vi "Accel_Read.vi"(8 "error in":errorcluster, 9 "Sensitivity":dbl, 10 "Axis":T3 items=["X-Axis", "Y-Axis", "Z-Axis"], 11 "I2CDevRef":T1 {"Device Address" format="%.0x"}) -> (0 "error out":errorcluster, 2 "Acceleration":dbl, 3 "I2CDevRef Out":T1 {"Device Address" format="%.0x"})   [LabVIEW 2011]
uses:
  Accel_ Axis.ctl
  <vilib>/Rock Robotics/WPI/I2C/WPI_I2CDevRef.ctl
  <vilib>/Rock Robotics/SystemInterfaces/Typedef/FPGA_TypedefDigitalModule.ctl
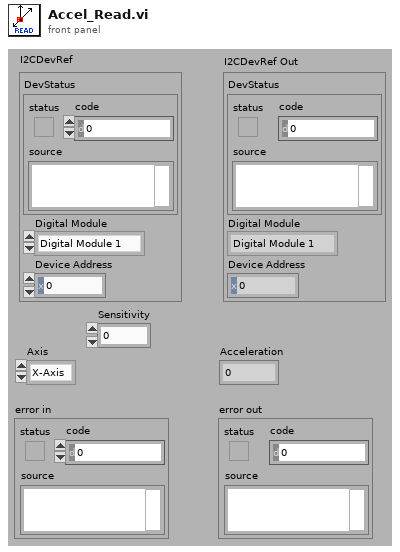
[diagram p1: front panel]
types:
  T1 = typedef "WPI_I2CDevRef.ctl" = cluster{"DevStatus":errorcluster, "Digital Module":T2, "Device Address":u8}
  T2 = typedef "FPGA_TypedefDigitalModule.ctl" = enum16{"Digital Module 1", "Digital Module 2"}
  T3 = typedef "Accel_ Axis.ctl" = u8
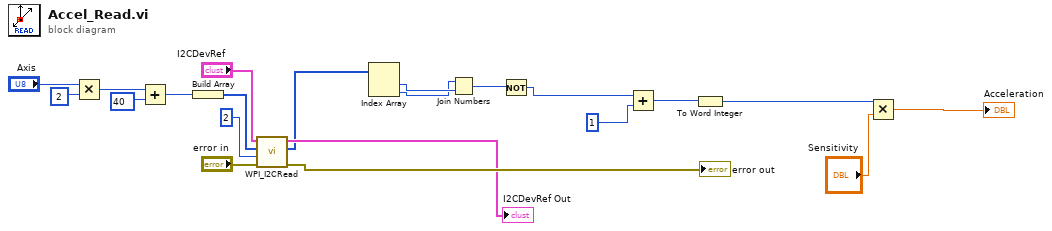
[diagram p0: block diagram]
diagram:
  n1 = Multiply(x="Axis", y=u8 2 ("Data To Send")) -> (x*y=w21:T3)
  n2 = Add(x=w21, y=u8 40 ("Data To Send")) -> (x+y=w11:T3)
  n3 = Build Array(w11) -> (w15:T3[])
  n4 = call <vilib>:"WPI_I2CRead.vi"("error in (no error)"="error in", "I2CBytesToRead"=u8 2, "I2CRegister"=w15, "I2CDevRef"="I2CDevRef") -> ("error out"=→"error out":errorcluster, "Data Out"=w7:u8[], "I2CDevRef"=→"I2CDevRef Out":T1)  [unwired: 1 in, 4 out]
  n5 = Index Array(array=w7) -> (element #1=w6:u8, element #2=w5:u8)  [unwired: 2 in]
  n6 = Join Numbers(hi=w5, lo=w6) -> ((hi.lo)=w4:u16)
  n7 = Not(x=w4) -> (.not. x?=w3:u16)
  n8 = Add(x=w3, y=1) -> (x+y=w2:i32)
  n9 = To Word Integer(number=w2) -> (16bit integer=w1:i16)
  n10 = Multiply(x=w1, y="Sensitivity") -> (x*y=→"Acceleration":dbl)
